vi "ANDOR_CheckTemp.vi"(7 "Set Temperatur":bool, 8 "error in (no error)":errorcluster, 11 "Temperature In":i32) -> (0 "error out":errorcluster, 2 "Stabilized?":bool, 3 "Temperature Out":sgl)   [LabVIEW 2010]
uses:
  <userlib>/_andor/atmcd32d.llb/Error Code Enum typedef.ctl
  <userlib>/_andor/atmcd32d.llb/FanMode_mode typedef.ctl
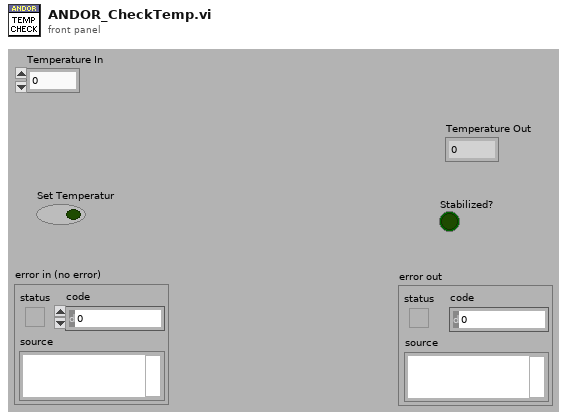
[diagram p1: front panel]
types:
  T1 = typedef "Error Code Enum typedef.ctl" = enum32{"N/A (0)", "DRV_ERROR_CODES", "DRV_SUCCESS", "DRV_VXDNOTINSTALLED", "DRV_ERROR_SCAN", "DRV_ERROR_CHECK_SUM", "DRV_ERROR_FILELOAD", "DRV_UNKNOWN_FUNC", "DRV_ERROR_VXD_INIT", "DRV_ERROR_ADDRESS", "DRV_ERROR_PAGELOCK", "DRV_ERROR_PAGEUNLOCK", "DRV_ERROR_BOARDTEST", "DRV_ERROR_ACK", "DRV_ERROR_UP_FIFO", "DRV_ERROR_PATTERN", "N/A (16)", "DRV_ACQUISITION_ERRORS", "DRV_ACQ_BUFFER", "DRV_ACQ_DOWNFIFO_FULL", "DRV_PROC_UNKONWN_INSTRUCTION", "DRV_ILLEGAL_OP_CODE", "DRV_KINETIC_TIME_NOT_MET", "DRV_ACCUM_TIME_NOT_MET", "DRV_NO_NEW_DATA", "N/A (25)", "DRV_SPOOLERROR", "N/A (27)", "N/A (28)", "N/A (29)", "N/A (30)", "N/A (31)", "N/A (32)", "DRV_TEMPERATURE_CODES", "DRV_TEMPERATURE_OFF", "DRV_TEMPERATURE_NOT_STABILIZED", "DRV_TEMPERATURE_STABILIZED", "DRV_TEMPERATURE_NOT_REACHED", "DRV_TEMPERATURE_OUT_RANGE", "DRV_TEMPERATURE_NOT_SUPPORTED", "DRV_TEMPERATURE_DRIFT", "N/A (41)", "N/A (42)", "N/A (43)", "N/A (44)", "N/A (45)", "N/A (46)", "N/A (47)", "N/A (48)", "DRV_GENERAL_ERRORS", "DRV_INVALID_AUX", "DRV_COF_NOTLOADED", "DRV_FPGAPROG", "DRV_FLEXERROR", "DRV_GPIBERROR", "N/A (55)", "N/A (56)", "N/A (57)", "N/A (58)", "N/A (59)", "N/A (60)", "N/A (61)", "N/A (62)", "N/A (63)", "DRV_DATATYPE", "DRV_DRIVER_ERRORS", "DRV_P1INVALID", "DRV_P2INVALID", "DRV_P3INVALID", "DRV_P4INVALID", "DRV_INIERROR", "DRV_COFERROR", "DRV_ACQUIRING", "DRV_IDLE", "DRV_TEMPCYCLE", "DRV_NOT_INITIALIZED", "DRV_P5INVALID", "DRV_P6INVALID", "DRV_INVALID_MODE", "DRV_INVALID_FILTER", "DRV_I2CERRORS", "DRV_I2CDEVNOTFOUND", "DRV_I2CTIMEOUT", "DRV_P7INVALID", "N/A (84)", "N/A (85)", "N/A (86)", "N/A (87)", "N/A (88)", "N/A (89)", "DRV_IOCERROR", "DRV_VRMVERSIONERROR"}
  T2 = typedef "FanMode_mode typedef.ctl" = enum16{"fan on full", "fan on low", "fan off"}
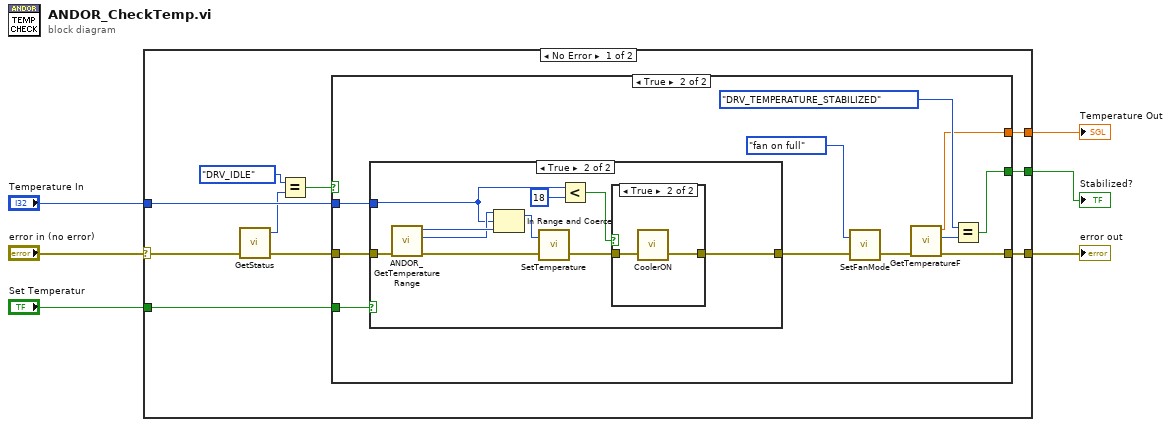
[diagram p0: block diagram]
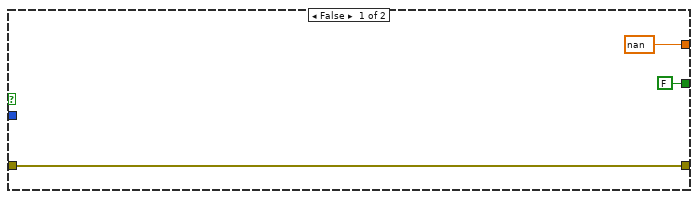
[diagram p2: hidden frame]
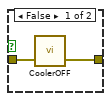
[diagram p4: hidden frame]
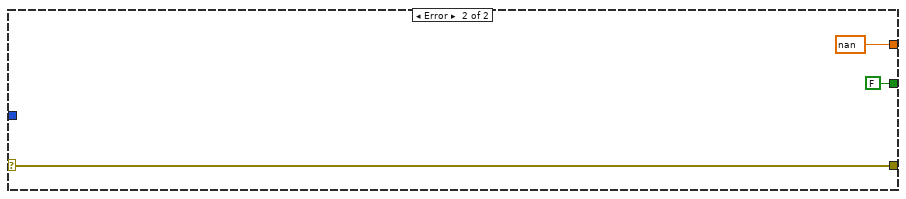
[diagram p5: hidden frame]
diagram:
  n1 = case shown="No Error" "error in (no error)" {
    selector: "error in (no error)" -> [w9 w48]
    tunnel: "Temperature In" -> [w16 _]
    tunnel: [w15 w48] -> w6
    tunnel: "Set Temperatur" -> [w14 _]
    tunnel: [w13 sgl nan] -> w3
    tunnel: [w12 FALSE] -> w2
    frame No Error {
      n2 = call <userlib>:"GetStatus.vi"("error in (no error)"=w9) -> ("error out"=w7:errorcluster, "status"=w11:T1)  [unwired: 2 in, 1 out]
      n3 = Equal?(x=Error_Code_Enum_typedef."DRV_IDLE" ("status"), y=w11) -> (x = y?=w8:bool)
      n4 = case shown="True" w8 {
        tunnel: w16 -> [_ w30]
        tunnel: [w19 w20] -> w15
        tunnel: w14 -> [_ w28]
        tunnel: [sgl nan w22] -> w13
        tunnel: [FALSE w25] -> w12
        tunnel: w7 -> [w19 w24]
        frame False {
        }
        frame True {
          n5 = case shown="True" w28 {
            tunnel: w30 -> [_ w32]
            tunnel: w24 -> [w31 w41]
            tunnel: [w31 w33] -> w29
            frame False {
            }
            frame True {
              n6 = call "ANDOR_GetTemperatureRange.vi"("error in (no error)"=w41) -> ("error out"=w40:errorcluster, "maxTemp"=w38:i32, "minTemp"=w39:i32)  [unwired: 6 in, 2 out]
              n7 = In Range and Coerce(upper limit=w38, x=w32, lower limit=w39) -> (coerced(x)=w37:i32)  [unwired: 1 out]
              n8 = call <userlib>:"SetTemperature.vi"("error in (no error)"=w40, "temperature"=w37) -> ("error out"=w34:errorcluster)  [unwired: 1 out]
              n9 = Less?(x=w32, y=18) -> (x < y?=w35:bool)
              n10 = case shown="True" w35 {
                tunnel: w34 -> [w43 w45]
                tunnel: [w42 w44] -> w33
                frame False {
                  n11 = call <userlib>:"CoolerOFF.vi"("error in (no error)"=w43) -> ("error out"=w42:errorcluster)  [unwired: 1 in, 1 out]
                }
                frame True {
                  n12 = call <userlib>:"CoolerON.vi"("error in (no error)"=w45) -> ("error out"=w44:errorcluster)  [unwired: 1 in, 1 out]
                }
              }
            }
          }
          n13 = call <userlib>:"SetFanMode.vi"("error in (no error)"=w29, "mode"=FanMode_mode_typedef."fan on full") -> ("error out"=w23:errorcluster)  [unwired: 1 out]
          n14 = call <userlib>:"GetTemperatureF.vi"("error in (no error)"=w23) -> ("error out"=w20:errorcluster, "status"=w21:T1, "temperature"=w22:sgl)  [unwired: 3 in, 1 out]
          n15 = Equal?(x=Error_Code_Enum_typedef."DRV_TEMPERATURE_STABILIZED" ("status"), y=w21) -> (x = y?=w25:bool)
        }
      }
    }
    frame Error {
    }
  }
  "error out" <- w6
  "Temperature Out" <- w3
  "Stabilized?" <- w2
